vi "Logic Tree.vi"() -> ()   [LabVIEW 2017]
panel:
  in  "Field String":string
  out "Name of Play":string
  in  "RL":T1(ring)
  in  "RR":T2(ring)
  in  "LR":T3(ring)
  in  "LL":T4(ring)
  in  "Position":enum16{"1", "2", "3"}(ring)
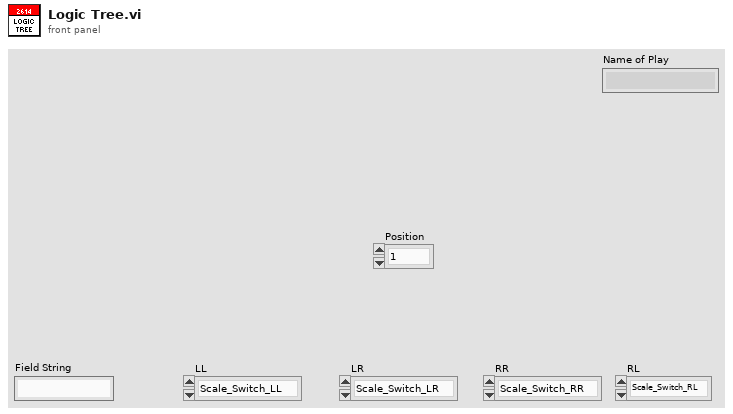
[diagram p1: front panel]
types:
  T1 = enum16{"Scale_Switch_RL", "Switch_Scale_RL", "Switch_2_RL", "Scale_2_RL", "Auto_Run_RL", "No_Op"}
  T2 = enum16{"Scale_Switch_RR", "Switch_Scale_RR", "Switch_2_RR", "Scale_2_RR", "Auto_Run_RR", "No_Op"}
  T3 = enum16{"Scale_Switch_LR", "Switch_Scale_LR", "Switch_2_LR", "Scale_2_LR", "Auto_Run_LR", "No_Op"}
  T4 = enum16{"Scale_Switch_LL", "Switch_Scale_LL", "Switch_2_LL", "Scale_2_LL", "Auto_Run_LL", "No_Op"}
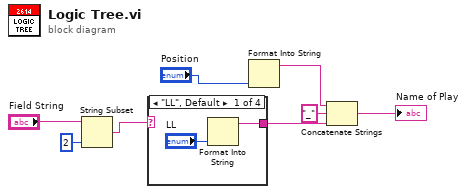
[diagram p0: block diagram]
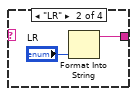
[diagram p2: hidden frame]
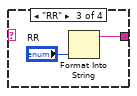
[diagram p3: hidden frame]
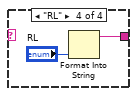
[diagram p4: hidden frame]
diagram:
  n1 = String Subset(string="Field String", length (rest)=2 ("length (rest)")) -> (substring=w3:string)  [unwired: 1 in]
  n2 = case shown="\"LL\", Default" w3 {
    tunnel: [w9 w12 w13 w15] -> w7
    frame "LL", Default {
      n3 = Format Into String("LL") -> (resulting string=w9:string)  [unwired: 3 in, 1 out]
    }
    frame "LR" {
      n4 = Format Into String("LR") -> (resulting string=w12:string)  [unwired: 3 in, 1 out]
    }
    frame "RR" {
      n5 = Format Into String("RR") -> (resulting string=w13:string)  [unwired: 3 in, 1 out]
    }
    frame "RL" {
      n6 = Format Into String("RL") -> (resulting string=w15:string)  [unwired: 3 in, 1 out]
    }
  }
  n7 = Format Into String("Position") -> (resulting string=w5:string)  [unwired: 3 in, 1 out]
  n8 = Concatenate Strings(w5, "_" ("string"), w7) -> (→"Name of Play":string)
